vi "Filter Logging.vi"(6 "Pauze?":bool, 8 "Data in":string[][](table), 9 "Searchtext":string, 10 "Column":u16, 11 "dup path":path) -> (0 "Unfiltered data out":string[][](array[string]), 3 "Filtered data out":string[][](table))   [LabVIEW 2012]
panel:
  out "text":string
  out "Timing (sec)":u32
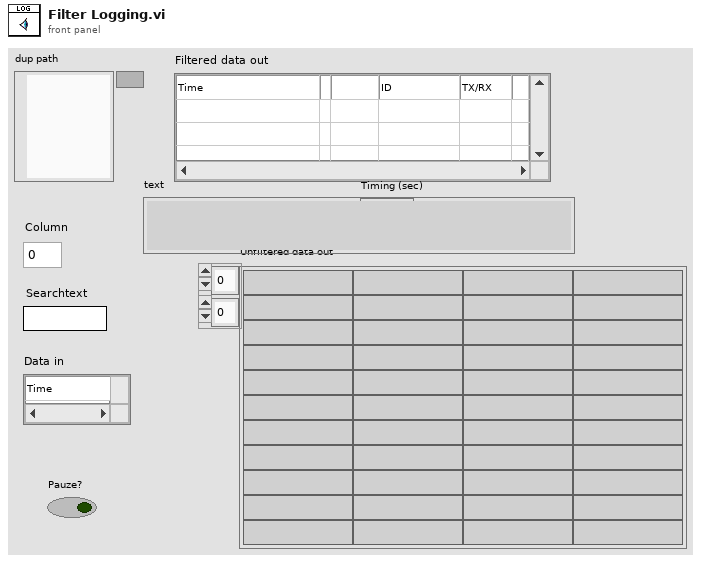
[diagram p1: front panel]
types:
  T1 = enum16{"open", "replace", "create", "open or create", "replace or create", "replace or create with confirmation"}
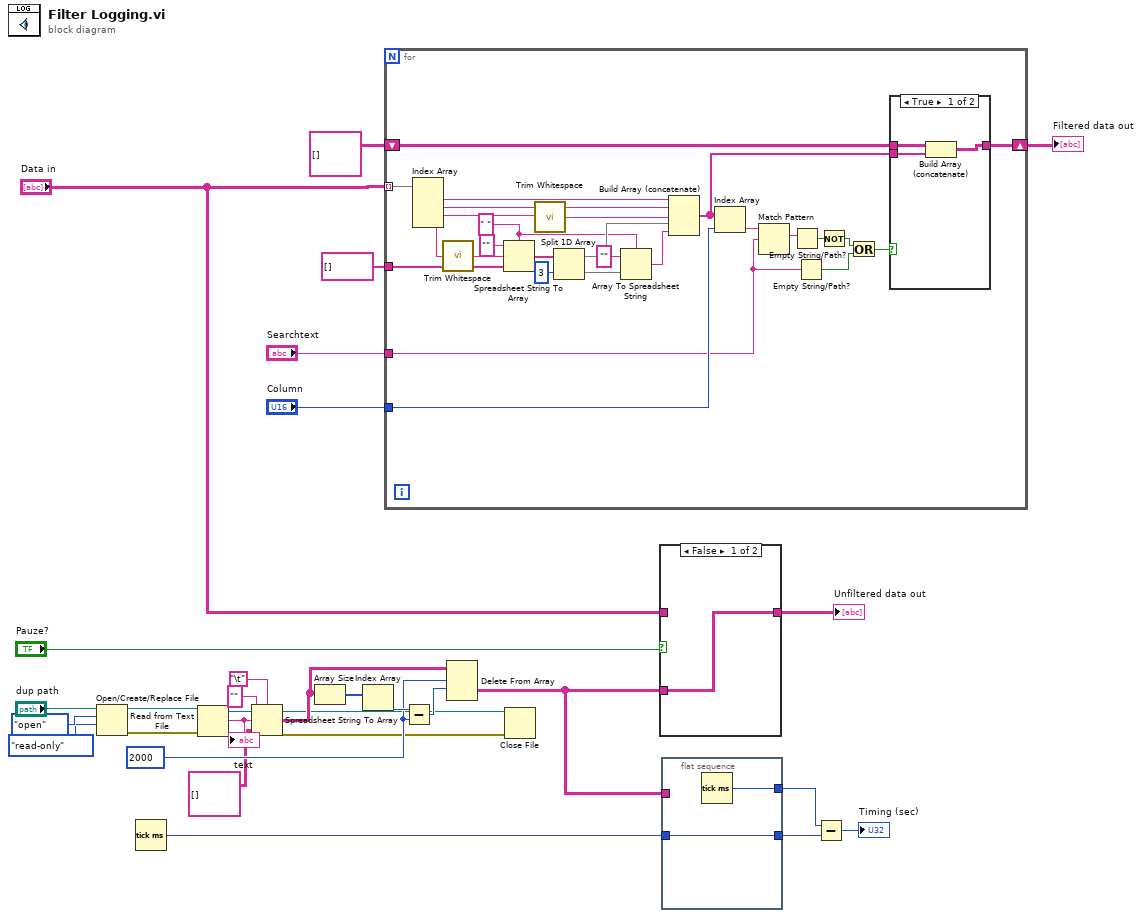
[diagram p0: block diagram]
diagram:
  w11 = 2000 ("y")
  n1 = Open/Create/Replace File(file path (use dialog)="dup path", operation (0:open)=T1."open", access (0:read/write)=enum16{"read/write", "read-only", "write-only"}."read-only") -> (refnum out=w2:refnum<file>, error out=w1:errorcluster)  [unwired: 3 in, 1 out]
  n2 = Tick Count (ms)() -> (millisecond timer value=w15:u32)
  n3 = Read from Text File(file (use dialog)=w2, error in=w1) -> (refnum out=w4:refnum<file>, text=w10:string, error out=w3:errorcluster)  [unwired: 2 in, 1 out]
  "text" <- w10
  n4 = Spreadsheet String To Array(delimiter (Tab)="\t", format string="", spreadsheet string=w10, array type (2D Dbl)=string[][] [] ("all rows")) -> (array=w7:string[][])
  n5 = Array Size(array=w7) -> (size(s)=w21:i32[])
  n6 = Index Array(array=w21) -> (element=w22:i32)  [unwired: 1 in]
  n7 = for {
    tunnel: "Data in" -> [w50] mode=indexing
    tunnel: string[] [] -> [w54]
    shift-right: [w39] -> w20
    shift-left: string[][] [] ("all rows") -> [w40]
    tunnel: "Column" -> [w42]
    tunnel: "Searchtext" -> [w36]
    w44 = " " ("delimiter (Tab)")
    n8 = Index Array(array=w50) -> (element #1=w56:string, element #2=w55:string, element #3=w31:string, element #4=w53:string)  [unwired: 4 in]
    n9 = call <vilib>:"Trim Whitespace.vi"("string"=w53) -> ("trimmed string"=w52:string)  [unwired: 1 in]
    n10 = Spreadsheet String To Array(delimiter (Tab)=w44, format string="", spreadsheet string=w52, array type (2D Dbl)=w54) -> (array=w49:string[])
    n11 = call <vilib>:"Trim Whitespace.vi"("string"=w31) -> ("trimmed string"=w30:string)  [unwired: 1 in]
    n12 = Split 1D Array(array=w49, index=3) -> (first subarray=w47:string[], second subarray=w46:string[])
    n13 = Array To Spreadsheet String(delimiter (Tab)=w44, array=w46, 3:"" ("format string")) -> (spreadsheet string=w45:string)
    n14 = Build Array (concatenate)(w56, w55, w30, w47, w45) -> (w38:string[])
    n15 = Index Array(array=w38, index=w42) -> (element=w41:string)
    n16 = Match Pattern(string=w41, regular expression=w36) -> (match substring=w37:string)  [unwired: 1 in, 3 out]
    n17 = Empty String/Path?(string/path=w37) -> (empty?=w33:bool)
    n18 = Empty String/Path?(string/path=w36) -> (empty?=w35:bool)
    n19 = Not(x=w33) -> (.not. x?=w32:bool)
    n20 = Or(x=w32, y=w35) -> (x .or. y?=w34:bool)
    n21 = case shown="True" w34 {
      tunnel: w40 -> [w59 w60]
      tunnel: [w57 w60] -> w39
      tunnel: w38 -> [w58 _]
      frame True {
        n22 = Build Array (concatenate)(w59, w58) -> (w57:string[][])
      }
      frame False {
      }
    }
  }
  "Filtered data out" <- w20
  n23 = Subtract(x=w22, y=w11) -> (x-y=w23:i32)
  n24 = Delete From Array(array=w7, length=w11, index (row)=w23) -> (deleted portion=w18:string[][])  [unwired: 1 in, 1 out]
  n25 = Close File(refnum=w4, error in=w3) -> ()  [unwired: 2 out]
  n26 = case shown="False" "Pauze?" {
    tunnel: [w61 w62] -> w25
    tunnel: "Data in" -> [_ w62]
    tunnel: w18 -> [w61 _]
    frame False {
    }
    frame True {
    }
  }
  "Unfiltered data out" <- w25
  n27 = flat-sequence {
    tunnel: w18 -> [_]
    tunnel: [w64] -> w17
    tunnel: [w63] -> w16
    tunnel: w15 -> [w63]
    frame #0 {
      n28 = Tick Count (ms)() -> (millisecond timer value=w64:u32)
    }
  }
  n29 = Subtract(x=w17, y=w16) -> (x-y=→"Timing (sec)":u32)
